vi "CountAt2DIndexNow_subvi.vi"(6 "Rounded Y Array":dbl[](array[numeric]), 7 "Index Y":i32, 9 "Rounded X Array":dbl[](array[numeric]), 10 "Index X":i32, 11 "Bin 2D array in":dbl[][](array[numeric])) -> (3 "Bin 2D array out":dbl[][](array[numeric]))   [LabVIEW 2019]
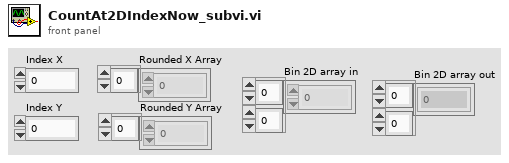
[diagram p1: front panel]
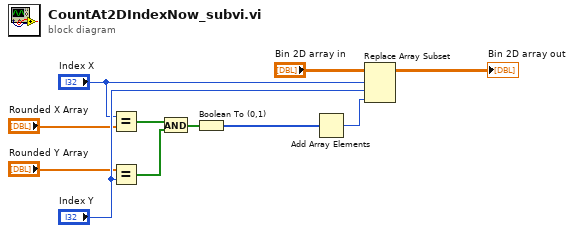
[diagram p0: block diagram]
diagram:
  n1 = Equal?(x="Index X", y="Rounded X Array") -> (x = y?=w2:bool[])
  n2 = Equal?(x="Rounded Y Array", y="Index Y") -> (x = y?=w5:bool[])
  n3 = And(x=w2, y=w5) -> (x .and. y?=w3:bool[])
  n4 = Boolean To (0,1)(Boolean=w3) -> (0, 1=w6:i16[])
  n5 = Add Array Elements(numeric array=w6) -> (sum=w9:i16)
  n6 = Replace Array Subset "Replace Array Subset"(array="Bin 2D array in", new element=w9, index (row)="Index X", index (col)="Index Y") -> (→"Bin 2D array out":dbl[][])
